vi "Service Micro.vi"(8 "error in (no error)":errorcluster, 10 "Caracter":string, 11 "Hardware in":refnum<class "Hardware.lvclass">) -> (0 "error out":errorcluster, 3 "Hardware out":refnum<class "Hardware.lvclass">)   [LabVIEW 2020, in "Hardware.lvlib" / "Hardware.lvclass"]
uses:
  Hardware.lvclass
  <vilib>/Instr/_visa.llb/VISA Configure Serial Port (Instr).vi
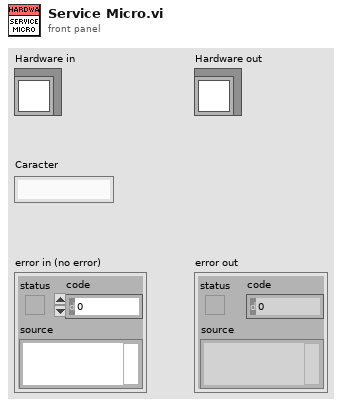
[diagram p1: front panel]
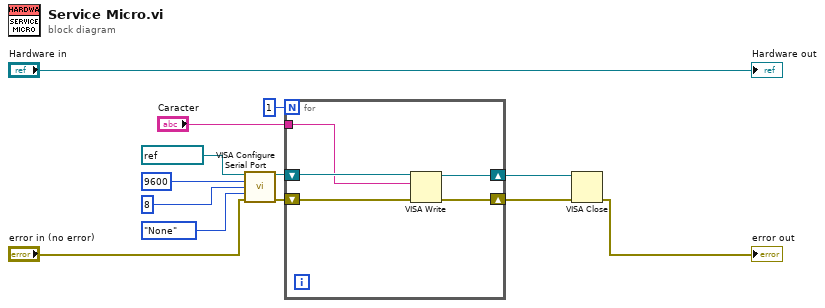
[diagram p0: block diagram]
diagram:
  n1 = call-poly "VISA Configure Serial Port"("VISA resource name"=refnum<visa-resource-name> "COM5", "baud rate (9600)"=u32 9600, "data bits (8)"=u16 8, "parity (0:none)"=enum16{"None", "Odd", "Even", "Mark", "Space"}."None", "error in (no error)"="error in (no error)") -> ("VISA resource name out"=w4:refnum<visa-resource-name>, "error out"=w6:errorcluster)  [unwired: 9 in]
  n2 = for {
    N: 1 -> [_]
    shift-right: [w18] -> w7
    shift-left: w6 -> [w17]
    shift-right: [w15] -> w3
    shift-left: w4 -> [w16]
    tunnel: "Caracter" -> [w14]
    n3 = VISA Write(VISA resource name=w16, write buffer=w14, error in (no error)=w17) -> (VISA resource name out=w15:refnum<visa-resource-name>, error out=w18:errorcluster)  [unwired: 1 out]
  }
  n4 = VISA Close(VISA resource name=w3, error in (no error)=w7) -> (error out=→"error out":errorcluster)
  "Hardware out" <- "Hardware in"
